vi "計算機.vi"() -> ()   [LabVIEW 2019]
panel:
  in  "stop":bool
  in  "Enum":enum16{"+", "\"-\"", "*", "/"}(ring)
  out "Numeric 3":dbl
  in  "Numeric 2":i64 min=0 max=100
  in  "Numeric":i64 format="%.0g"
  # "="
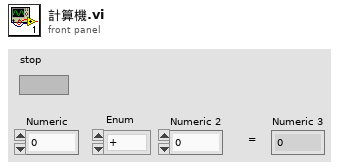
[diagram p1: front panel]
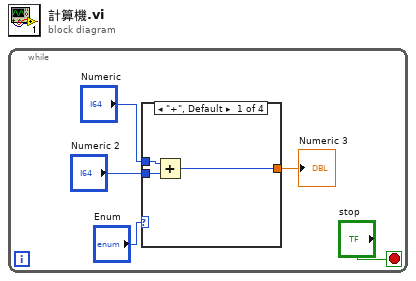
[diagram p0: block diagram]
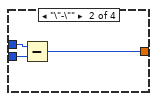
[diagram p2: hidden frame]
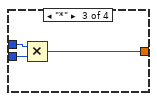
[diagram p3: hidden frame]
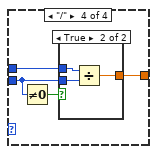
[diagram p4: hidden frame]
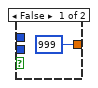
[diagram p5: hidden frame]
diagram:
  n1 = while {
    stop <- "stop" stop-if-true
    n2 = case shown="\"+\", Default" "Enum" {
      tunnel: "Numeric" -> [w8 w11 w14 w18]
      tunnel: [w7 w10 w13 w17] -> w3
      tunnel: "Numeric 2" -> [w6 w9 w12 w15]
      frame "+", Default {
        n3 = Add(x=w8, y=w6) -> (x+y=w7:i64)
      }
      frame "\"-\"" {
        n4 = Subtract(x=w11, y=w9) -> (x-y=w10:i64)
      }
      frame "*" {
        n5 = Multiply(x=w14, y=w12) -> (x*y=w13:i64)
      }
      frame "/" {
        n6 = Not Equal To 0?(x=w15) -> (x != 0?=w16:bool)
        n7 = case shown="True" w16 {
          tunnel: w18 -> [_ w22]
          tunnel: [999 w21] -> w17
          tunnel: w15 -> [_ w20]
          frame False {
          }
          frame True {
            n8 = Divide(x=w22, y=w20) -> (x/y=w21:dbl)
          }
        }
      }
    }
    "Numeric 3" <- w3
  }
